vi "AmplitudeModulation_2022.vi"() -> ()   [LabVIEW 2015]
uses:
  <vilib>/Platform/TimedLoop/XDataNode/timing_clust.ctl
  <vilib>/Platform/TimedLoop/XDataNode/nitl_modes.ctl
  <vilib>/Platform/TimedLoop/XDataNode/wakeup.ctl
  <vilib>/DAQmx/read.llb/DAQmx Read (Analog 1D DBL NChan 1Samp).vi
  <vilib>/DAQmx/miscellaneous.llb/DAQmx Fill In Error Info.vi
  <vilib>/addons/control/pid/pid.llb/PID (DBL).vi
  <vilib>/platform/TimedLoop/XDataNode/XDataNode.xnode
  <instrlib>/Agilent 33XXX Series/Agilent 33XXX Series.lvlib
  <vilib>/addons/control/pid/NI_PID_pid.lvlib
  <vilib>/Platform/TimedLoop/XDataNode/XDNodeRunTimeDep.lvlib
panel:
  in  "View Saved Data\nUpon Completion":bool
  out "Time Elapsed (s)":u32
  out "Temperature":dbl[](graph) caption="Signals"
  in  "Slide":dbl(slide) scale=35.0..45.0
  in  "Start":bool
  in  "Feed back Mechanism":enum32{"PID Control", "Simple P Control"}(tab)
  in  "PID gains":T1={"proportional gain (Kc)"=0.03, "integral time (Ti, min)"=0.175, "derivative time (Td, min)"=0.001} {"derivative time (Td, min)" format="%.3f"; "integral time (Ti, min)" format="%.3f"; "proportional gain (Kc)" format="%.3f"}
  in  "Simple P":dbl
  in  "Amplitude\nModulation?":bool=TRUE
  in  "voltage limit":dbl=0.15 format="%#_13g"
  in  "Set Point (C)":dbl=42.0
  in  "Total Time (s)":u32=300
  in  "Output":bool=TRUE
  in  "Amplitude (V)":dbl=0.01 format="%#_3g"
  in  "Stop":bool
  out "Current Reading":dbl=23.993355509891316 format="%#.1g"
  out "Waveform Chart":waveform(dbl)(graph)={"t0"=timestamp(3753893587.480759 s since 1904-01-01), "dt"=0.25, "Y"=[24.003649480079382, 24.007080753730627, 24.007080753730627, 24.007080753730627, 24.007080753730627, 24.01051200251053, 24.01051200251053, 24.003649480079382, 24.003649480079382, 24.007080753730627, 24.01051200251053, 24.007080753730627, 24.007080753730627, 24.003649480079382, 24.00021818155617, 24.003649480079382, 24.003649480079382, 24.00021818155617, 24.00021818155617, 23.99678685816036, 23.993355509891316, 23.99678685816036, 23.993355509891316]}
  in  "Log Data?":bool=TRUE
  in  "Description":string="Test Data. See Pictures."
  in  "File Path":path=path "C:/Data/Sonify Labview/2022/12192022/Pork-5Min-42C.lvm" caption="Filename"
  # "(Set Point - Current Reading) * P\n+ Current Voltage\n= New Voltage"
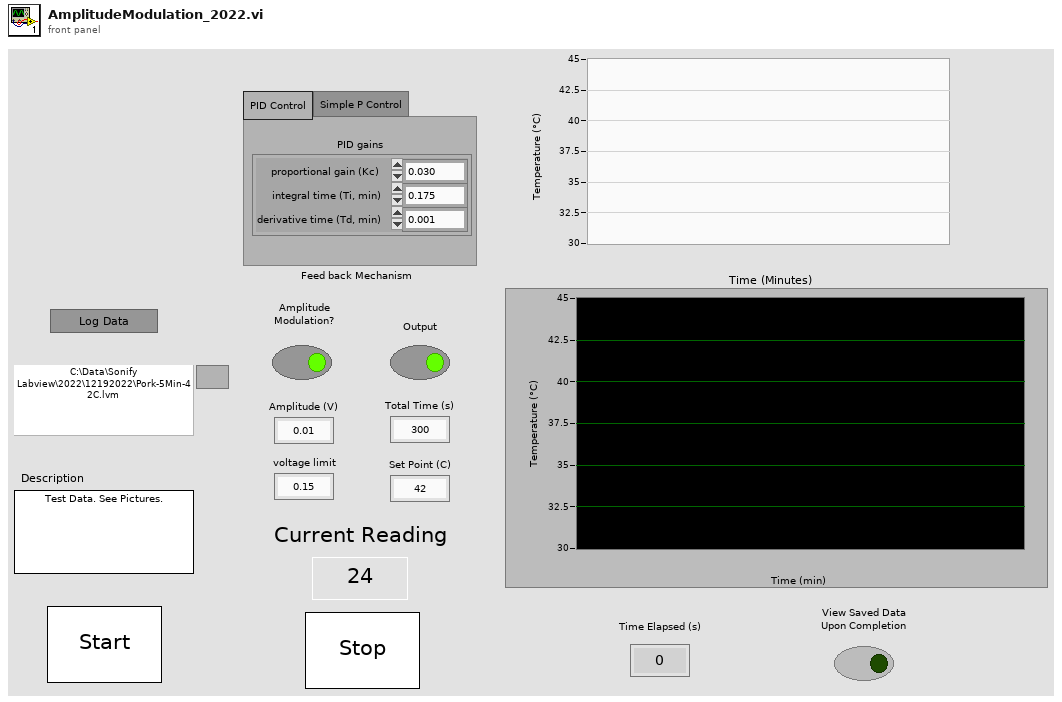
[diagram p1: front panel]
types:
  T1 = cluster{"proportional gain (Kc)":dbl, "integral time (Ti, min)":dbl, "derivative time (Td, min)":dbl}
  T2 = typedef "XDNodeRunTimeDep.lvlib/timing_clust.ctl" = cluster{"Expected End [f-1]":u64, "Actual End [f-1]":u64, "Finished Late? [f-1]":bool, "Expected End [i-1]":u64, "Actual End [i-1]":u64, "Finished Late? [i-1]":bool, "Expected Start [i]":u64, "Actual Start [i]":u64, "Expected Start [f]":u64, "Actual Start [f]":u64, "Source Name":string, "Structure Name":string, "Period":i64, "Deadline":i64, "Offset":i64, "Start":i64, "Priority":i32, "Timeout":i32, "Mode":T3, "Wakeup Reason":T4, "Error":errorcluster, "Source Type":string, "Secondary Source Type":string, "Global End Time":u64, "Global Start Time":u64, "Frame Duration":u64, "Iteration Duration":u64, "Assigned CPU":i32, "I/O Scan Engine Mode":u32}
  T3 = typedef "XDNodeRunTimeDep.lvlib/nitl_modes.ctl" = enum32{"No Change", "Process missed periods, maintain original phase", "Discard missed periods, maintain original phase", "Process missed periods, ignore original phase", "Discard missed periods, ignore original phase"}
  T4 = typedef "XDNodeRunTimeDep.lvlib/wakeup.ctl" = enum32{"Normal", "Aborted", "Asynchronous wakeup", "Timing source error", "Timed loop error", "Timeout"}
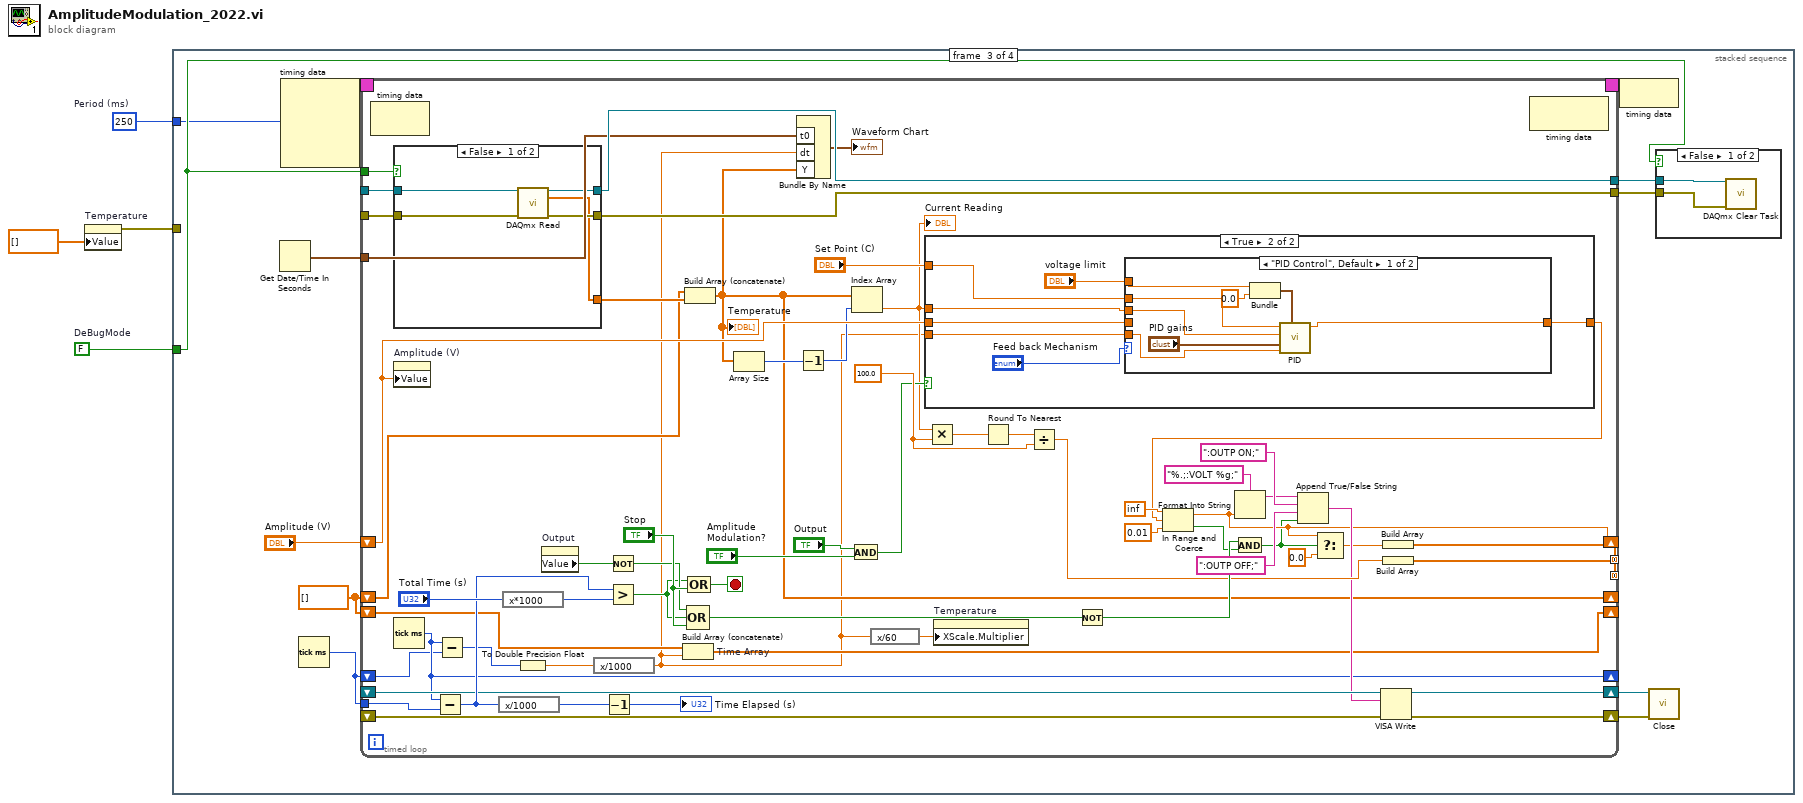
[diagram p0: block diagram]
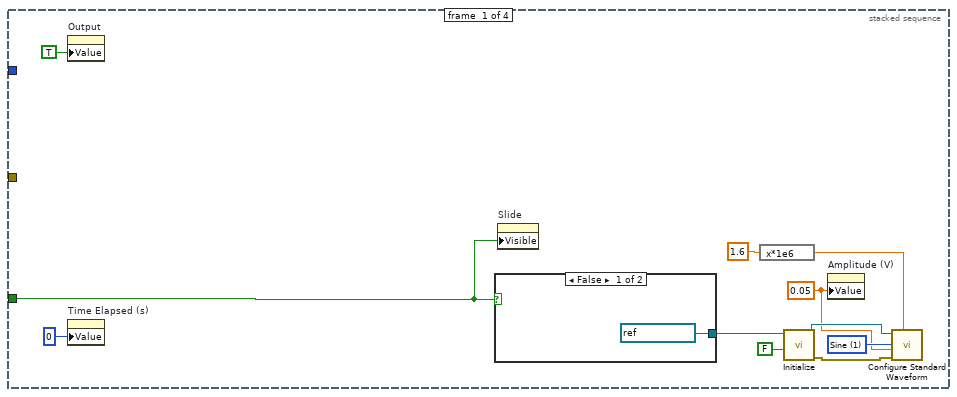
[diagram p2: hidden frame]
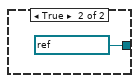
[diagram p3: hidden frame]
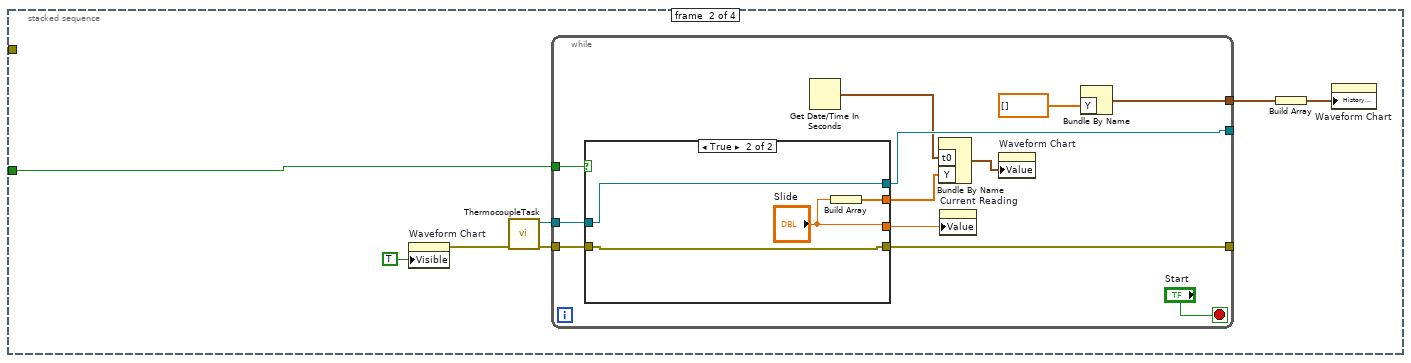
[diagram p4: hidden frame]
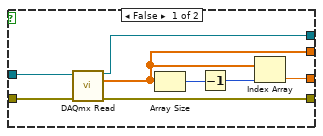
[diagram p5: hidden frame]
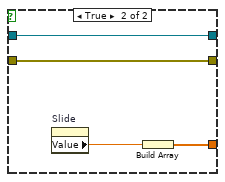
[diagram p6: hidden frame]
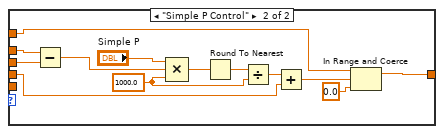
[diagram p8: hidden frame]
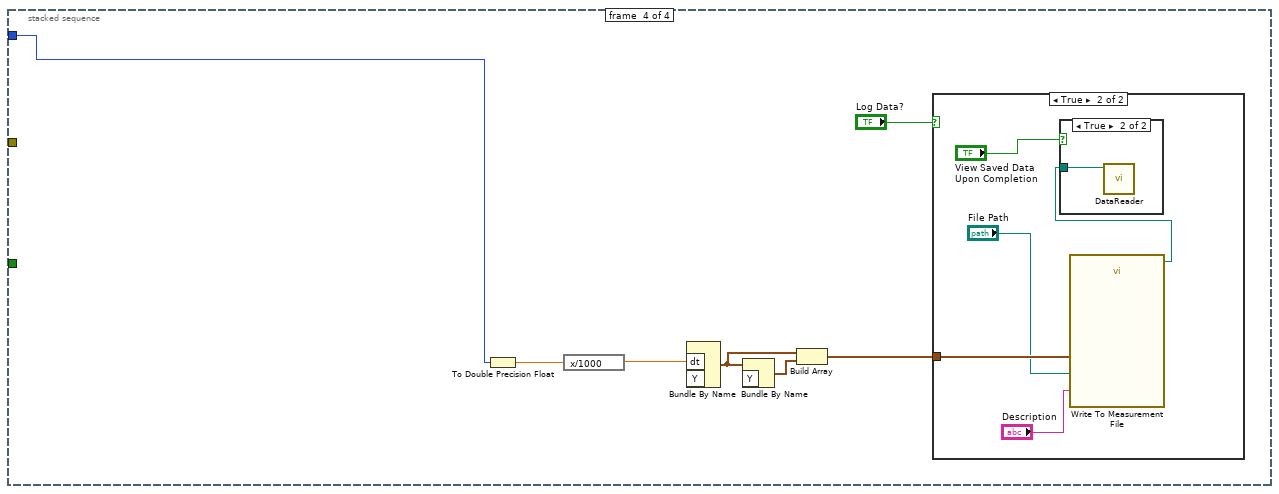
[diagram p10: hidden frame]
diagram:
  w1 = i64 250  # Period (ms)
  w4 = FALSE  # DeBugMode
  n1 = property on="Temperature" class="WFGraph (strict)"("Value"=dbl[] []) -> (error out=w3:errorcluster)  [unwired: 2 in, 1 out]
  n2 = stacked-sequence {
    seq-local: [_ _ w68 _] -> [_ _ _ w186]
    seq-local: [w9 _ _ _] -> [_ _ w64 _]
    seq-local: [w8 _ _ _] -> [_ _ w63 _]
    seq-local: [_ w26 _ _] -> [_ _ w61 _]
    seq-local: [_ w25 _ _] -> [_ _ w57 _]
    seq-local: [_ _ w60 _] -> [_ _ _ w185]
    tunnel: w4 -> [w5 w22 w59 _]
    tunnel: w3 -> [_ _ _ _]
    tunnel: w1 -> [_ _ w53 w179]
    frame #0 {
      w11 = u16 1 items=["DC", "Sine", "Square", "Triangle", "Ramp", "Pulse", "Noise", "Sinc", "Negative Ramp", "Exponential Rise", "Exponential Fall", "Cardiac"] ("Waveform Function (1: Sine)")
      w6 = 0.05 ("Amplitude (1)")
      n3 = property on="Output" class="Bool (strict)"("Value"=TRUE ("Enable Output  (T: Enable)")) -> ()  [unwired: 2 in, 2 out]
      n4 = property on="Time Elapsed (s)" class="DigNum (strict)"("Value"=u32 0 ("Time Elapsed (s)")) -> ()  [unwired: 2 in, 2 out]
      n5 = case shown="False" w5 {
        tunnel: [refnum<visa-resource-name> "FunGen1" ("Function Gen Address") refnum<visa-resource-name> "FunGen2" ("Function Gen Address")] -> w15
        frame False {
        }
        frame True {
        }
      }
      n6 = property on="Slide" class="Slide (strict)"("Visible"=w5) -> ()  [unwired: 2 in, 2 out]
      n7 = expression code="x*1e6"(1.6 ("Frequency (1000 Hz)")) -> (w7:dbl)
      n8 = call <instrlib>:"Initialize.vi"("Reset (True)"=FALSE, "VISA resource name"=w15) -> ("error out"=w13:errorcluster, "VISA resource name out"=w14:refnum<visa-resource-name>)  [unwired: 8 in]
      n9 = property on="Amplitude (V)" class="DigNum (strict)"("Value"=w6) -> ()  [unwired: 2 in, 2 out]
      n10 = call <instrlib>:"Configure Standard Waveform.vi"("Frequency (1000 Hz)"=w7, "error in (no error)"=w13, "Amplitude (1)"=w6, "Waveform Function (1: Sine)"=w11, "VISA resource name"=w14) -> ("error out"=w8:errorcluster, "VISA resource name out"=w9:refnum<visa-resource-name>)  [unwired: 5 in]
    }
    frame #1 {
      n11 = property on="Waveform Chart" class="WFChart (strict)"("Visible"=TRUE) -> (error out=w20:errorcluster)  [unwired: 2 in, 1 out]
      n12 = call "ThermocoupleTask.vi"("error in"=w20) -> ("error out"=w27:errorcluster, "task out"=w28:refnum<k21>)  [unwired: 9 in]
      n13 = while {
        tunnel: w28 -> [w40]
        tunnel: w27 -> [w39]
        tunnel: [w35] -> w26
        tunnel: [w34] -> w25
        tunnel: [w32] -> w24
        tunnel: w22 -> [w30]
        stop <- "Start" stop-if-true
        n14 = case shown="True" w30 {
          tunnel: w40 -> [w48 w52]
          tunnel: w39 -> [w47 w51]
          tunnel: [w44 w49] -> w37
          tunnel: [w43 "Slide"] -> w36
          tunnel: [w42 w52] -> w35
          tunnel: [w41 w51] -> w34
          frame False {
            n15 = call-poly <vilib>:"DAQmx Read.vi"("task/channels in"=w48, "error in"=w47) -> ("task out"=w42:refnum<k21>, "data"=w44:dbl[], "error out"=w41:errorcluster)  [unwired: 11 in]
            n16 = Array Size(array=w44) -> (size(s)=w46:i32)
            n17 = Decrement(x=w46) -> (x-1=w45:i32)
            n18 = Index Array(array=w44, index=w45) -> (element=w43:dbl)
          }
          frame True {
            n19 = Build Array("Slide") -> (w49:dbl[])
          }
        }
        n20 = Get Date/Time In Seconds() -> (seconds since 1Jan1904=w29:timestamp)
        n21 = Bundle By Name("t0"=w29, "Y"=w37) -> (w33:waveform(dbl))  [unwired: 1 in]
        n22 = property on="Current Reading" class="DigNum (strict)"("Value"=w36) -> ()  [unwired: 2 in, 2 out]
        n23 = property on="Waveform Chart" class="WFChart (strict)"("Value"=w33) -> ()  [unwired: 2 in, 2 out]
        n24 = Bundle By Name("Y"=dbl[] []) -> (w32:waveform(dbl))  [unwired: 1 in]
      }
      n25 = Build Array(w24) -> (w23:waveform(dbl)[])
      n26 = property on="Waveform Chart" class="WFChart (strict)"("History Data"=w23) -> ()  [unwired: 2 in, 2 out]
    }
    frame #2 {
      w56 = dbl[] []
      n27 = Get Date/Time In Seconds() -> (seconds since 1Jan1904=w58:timestamp)
      n28 = node-c288(w53) -> (w55:T2)  [unwired: 3 in]
      n29 = Tick Count (ms)() -> (millisecond timer value=w65:u32)
      n30 = timed-loop {
        shift-right: [w109] -> w70
        shift-left: w63 -> [w107]
        shift-right: [w110] -> w69
        shift-left: w64 -> [w108]
        tunnel: w65 -> [w100]
        shift-right: [w85] -> _
        shift-left: "Amplitude (V)" -> [w106]
        tunnel: [w124] -> w68 mode=concatenating
        shift-right: [w92] -> _
        shift-left: w65 -> [w91]
        tunnel: w61 -> [w96]
        tunnel: [w95] -> w67
        tunnel: [w94] -> w66
        tunnel: w57 -> [w93]
        tunnel: [w81] -> w60 mode=concatenating
        tunnel: w59 -> [w79]
        shift-right: [w76] -> _
        shift-left: w56 -> [w77]
        tunnel: w58 -> [w75]
        shift-right: [w73] -> _
        shift-left: w56 -> [w74]
        timing: w55 -> [_]
        timing-out: [_] -> w54
        stop <- w132 stop-if-true
        w120 = 100.0 ("y")
        n31 = node-c288() -> ()  [unwired: 1 in, 1 out]
        n32 = case shown="False" w79 {
          tunnel: w96 -> [w139 w141]
          tunnel: [w138 w141] -> w95
          tunnel: [w137 w140] -> w94
          tunnel: w93 -> [w136 w140]
          tunnel: [w135 w142] -> w78
          frame False {
            n33 = call-poly <vilib>:"DAQmx Read.vi"("task/channels in"=w139, "error in"=w136) -> ("task out"=w138:refnum<k21>, "data"=w135:dbl[], "error out"=w137:errorcluster)  [unwired: 11 in]
          }
          frame True {
            n34 = property on="Slide" class="Slide (strict)"() -> ("Value"=w143:dbl)  [unwired: 2 in, 2 out]
            n35 = Build Array(w143) -> (w142:dbl[])
          }
        }
        n36 = property on="Amplitude (V)" class="DigNum (strict)"("Value"=w106) -> ()  [unwired: 2 in, 2 out]
        n37 = Tick Count (ms)() -> (millisecond timer value=w92:u32)
        n38 = Subtract(x=w92, y=w100) -> (x-y=w112:u32)
        n39 = Subtract(x=w92, y=w91) -> (x-y=w90:u32)
        n40 = expression code="x/1000"(w112) -> (w87:u32)
        n41 = expression code="x*1000"("Total Time (s)") -> (w130:u32)
        n42 = To Double Precision Float(number=w90) -> (double precision float=w89:dbl)
        n43 = property on="Output" class="Bool (strict)"() -> ("Value"=w126:bool)  [unwired: 2 in, 2 out]
        n44 = expression code="x/1000"(w89) -> (w71:dbl)
        n45 = Decrement(x=w87) -> (x-1=→"Time Elapsed (s)":u32)
        n46 = Not(x=w126) -> (.not. x?=w119:bool)
        n47 = Greater?(x=w112, y=w130) -> (0:w118:bool)
        n48 = Build Array (concatenate) "Time Array"(w74, w71) -> (w73:dbl[])
        n49 = Build Array (concatenate)(w77, w78) -> (w76:dbl[])
        "Temperature" <- w76
        n50 = Compound Arithmetic op=OR(w119, w118, "Stop") -> (w128:bool)
        n51 = Compound Arithmetic op=OR(w118, "Stop") -> (w132:bool)
        n52 = Array Size(array=w76) -> (size(s)=w98:i32)
        n53 = Bundle By Name("t0"=w75, "dt"=w71, "Y"=w76) -> (→"Waveform Chart":waveform(dbl))  [unwired: 1 in]
        n54 = Decrement(x=w98) -> (x-1=w97:i32)
        n55 = And(x="Output", y="Amplitude\nModulation?") -> (x .and. y?=w113:bool)
        n56 = Index Array(array=w76, index=w97) -> (element=w99:dbl)
        "Current Reading" <- w99
        n57 = expression code="x/60"(w71) -> (w72:dbl)
        n58 = case shown="True" w113 {
          tunnel: w99 -> [_ w150]
          tunnel: [w144 w148] -> w111
          tunnel: w106 -> [w144 w149]
          tunnel: "Set Point (C)" -> [_ w151]
          tunnel: w71 -> [_ w146]
          frame False {
          }
          frame True {
            n59 = case shown="\"PID Control\", Default" "Feed back Mechanism" {
              tunnel: w151 -> [w155 w169]
              tunnel: w150 -> [w153 w168]
              tunnel: w149 -> [_ w166]
              tunnel: [w156 w163] -> w148
              tunnel: "voltage limit" -> [w154 w165]
              tunnel: w146 -> [w152 _]
              frame "PID Control", Default {
                n60 = Bundle("voltage limit"=w154, "output low"=0.0) -> (w159:cluster{"voltage limit":dbl, "output low":dbl})  [unwired: 1 in]
                n61 = call-poly <vilib>:"PID.vi"("output range"=w159, "dt (s)"=w152, "PID gains"="PID gains", "process variable"=w153, "setpoint"=w155) -> ("output"=w156:dbl)  [unwired: 5 in, 1 out]
              }
              frame "Simple P Control" {
                w170 = 1000.0 ("y")
                n62 = Subtract(x=w169, y=w168) -> (x-y=w161:dbl)
                n63 = Compound Arithmetic op=MULTIPLY("Simple P", w161, w170) -> (w172:dbl)
                n64 = Round To Nearest(number=w172) -> (nearest integer value=w171:dbl)
                n65 = Divide(x=w171, y=w170) -> (x/y=w167:dbl)
                n66 = Add(x=w167, y=w166) -> (x+y=w164:dbl)
                n67 = In Range and Coerce(upper limit=w165, x=w164, lower limit=0.0) -> (coerced(x)=w163:dbl)  [unwired: 1 out]
              }
            }
          }
        }
        n68 = Multiply(x=w99, y=w120) -> (x*y=w123:dbl)
        n69 = property on="Temperature" class="WFGraph (strict)"("XScale.Multiplier"=w72) -> ()  [unwired: 2 in, 2 out]
        n70 = Round To Nearest(number=w123) -> (nearest integer value=w122:dbl)
        n71 = Divide(x=w122, y=w120) -> (x/y=w121:dbl)
        n72 = Not(x=w128) -> (.not. x?=w129:bool)
        n73 = In Range and Coerce(upper limit=inf, x=w111, lower limit=0.01) -> (coerced(x)=w85:dbl, In Range?=w114:bool)
        n74 = Format Into String(format string="%.;:VOLT %g;" ("Amplitude Command"), w85) -> (resulting string=w102:string)  [unwired: 2 in, 1 out]
        n75 = And(x=w129, y=w114) -> (x .and. y?=w83:bool)
        n76 = Append True/False String(1:w83, 2:":OUTP OFF;" ("true string"), 3:":OUTP ON;" ("true string"), 4:w102) -> (0:w101:string)
        n77 = Select(t=w85, s=w83, f=0.0) -> (s? t:f=w82:dbl)
        n78 = VISA Write(VISA resource name=w108, write buffer=w101, error in (no error)=w107) -> (VISA resource name out=w110:refnum<visa-resource-name>, error out=w109:errorcluster)  [unwired: 1 out]
        n79 = Build Array(w82) -> (w81:dbl[])
        n80 = Build Array(w121) -> (w124:dbl[])
        n81 = node-c288() -> ()  [unwired: 1 in, 1 out]
      }
      n82 = node-c288(w54) -> ()
      n83 = call <instrlib>:"Close.vi"("error in (no error)"=w70, "VISA resource name"=w69) -> ()  [unwired: 9 in, 1 out]
      n84 = case shown="False" w59 {
        tunnel: w67 -> [w178 _]
        tunnel: w66 -> [w177 _]
        frame False {
          n85 = call <vilib>:"DAQmx Clear Task.vi"("task in"=w178, "error in"=w177) -> ()  [unwired: 13 in, 1 out]
        }
        frame True {
        }
      }
    }
    frame #3 {
      n86 = To Double Precision Float(number=w179) -> (double precision float=w181:dbl)
      n87 = expression code="x/1000"(w181) -> (w180:dbl)
      n88 = Bundle By Name("dt"=w180, "Y"=w186) -> (w182:waveform(dbl))  [unwired: 1 in]
      n89 = Bundle By Name(cluster=w182, "Y"=w185) -> (w184:waveform(dbl))
      n90 = Build Array(w182, w184) -> (w183:waveform(dbl)[])
      n91 = case shown="True" "Log Data?" {
        tunnel: w183 -> [_ w191]
        frame False {
        }
        frame True {
          n92 = call "Write To Measurement File"("Signals"=w191, "Filename"="File Path", "Comment"="Description") -> ("Filename Out"=w188:path)  [unwired: 14 in, 2 out]
          n93 = case shown="True" "View Saved Data\nUpon Completion" {
            tunnel: w188 -> [_ w193]
            frame False {
            }
            frame True {
              n94 = call "DataReader.vi"("Filename"=w193) -> ()  [unwired: 11 in]
            }
          }
        }
      }
    }
  }
